vi "Set Pump State.vi"(8 "error in (no error)":cluster{"状态":bool, "代码":i32, "源":string} caption="错误输入（无错误）", 10 "泵状态":bool, 11 "硬件蒸发冷却器输入":refnum<class "HW Evaporative Cooler.lvclass">) -> (0 "error out":cluster{"状态":bool, "代码":i32, "源":string} caption="错误输出")   [LabVIEW 2015, in "HW Evaporative Cooler.lvclass"]
uses:
  HW Evaporative Cooler.lvclass
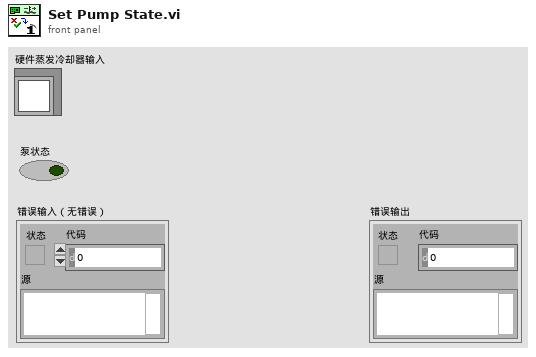
[diagram p1: front panel]
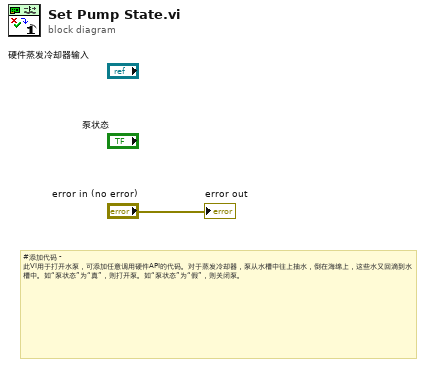
[diagram p0: block diagram]
diagram:
  # "#添加代码 - 此VI用于打开水泵，可添加任意调用硬件API的代码。对于蒸发冷却器，泵从水槽中往上抽水，倒在海绵上，这些水又回滴到水槽中。如“泵状态”为“真”，则打开泵。如“泵状态”为“假”，则关闭泵。"
  "error out" <- "error in (no error)"
